vi "Read Parameters from List.vi"(8 "error in (no error)":errorcluster, 11 "Scan SBlock in":refnum<class "Scan SBlock.lvclass">) -> (0 "error out":errorcluster, 2 "Parameters from List":T1[](array[typedef]), 3 "Scan SBlock out":refnum<class "Scan SBlock.lvclass">)   [LabVIEW 2020, in "Run Utilities.lvlib" / "Scan SBlock.lvclass"]
uses:
  Scan SBlock.lvclass
  Advanced Parameters - list.ctl
  Scan SBlock.lvclass/Scan SBlock.ctl
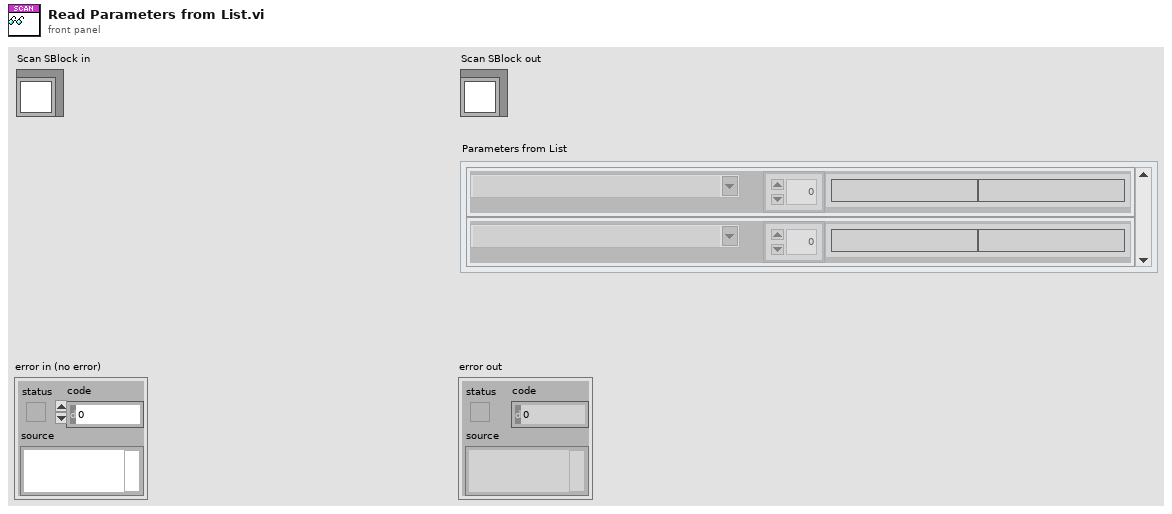
[diagram p1: front panel]
types:
  T1 = typedef "Run Utilities.lvlib/Scan SBlock.lvclass/Advanced Parameters - list.ctl" = cluster{"Param":string, "List of values":string[]}
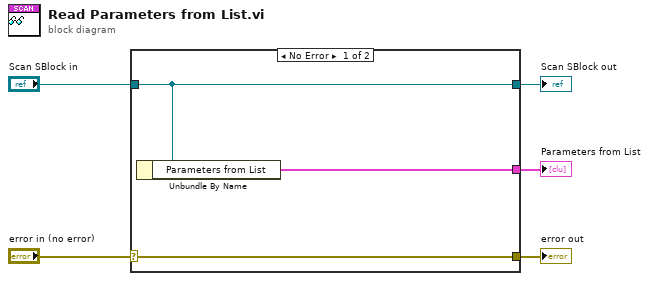
[diagram p0: block diagram]
diagram:
  n1 = case shown="No Error" "error in (no error)" {
    selector: "error in (no error)" -> [w8 w9]
    tunnel: [w8 w9] -> w4
    tunnel: [w7 w10] -> w2
    tunnel: "Scan SBlock in" -> [w7 w10]
    tunnel: [w6 _] -> w1
    frame No Error {
      n2 = Unbundle By Name(w7) -> ("Parameters from List"=w6:T1[])
    }
    frame Error {
    }
  }
  "error out" <- w4
  "Scan SBlock out" <- w2
  "Parameters from List" <- w1
